vi "GetClassPath.vi"(8 "error in":errorcluster, 10 "class name":string, 11 "CEF_Repository in":refnum<class "CEF_Repository.lvclass">) -> (0 "error out":errorcluster, 2 "class path":path, 3 "CEF_Repository out":refnum<class "CEF_Repository.lvclass">)   [LabVIEW 2023, in "CEF.lvlib" / "CEF_Repository.lvclass"]
doc: "Gets the path to the Class based on the Class Name. \nThe default behavior is build the path of the class on top of the class folder path. The name of the class and the folder it contains needs to be the same. A simple lookup from index and name would be the other option.\nCopyright 2017 National Instruments Corporation\n\nLicensed under the Apache License, Version 2.0 (the \"License\"); you may not use this file except in compliance with the License. You may obtain a copy of the License at http://www.apache.org/licenses/LICENSE-2.0\nUnless required by applicable law or agreed to in writing, software distributed under the License is distributed on an \"AS IS\" BASIS, WITHOUT WARRANTIES OR CONDITIONS OF ANY KIND, either express or implied. See the License for the specific language governing permissions and limitations under the License."
uses:
  CEF_Repository.lvclass
  class discovery singleton/class discovery singleton methods.ctl
  CEF.lvlib
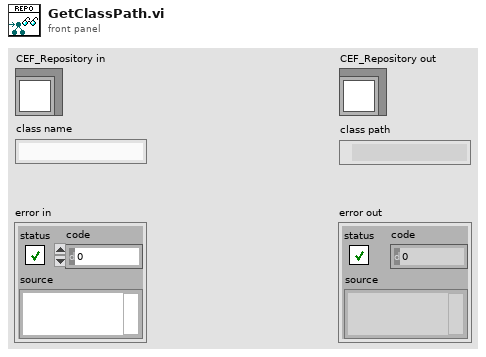
[diagram p1: front panel]
types:
  T1 = typedef "CEF.lvlib/class discovery singleton methods.ctl" = enum16{"add search paths", "load class by name", "list available classes", "get class path", "delete cache"}
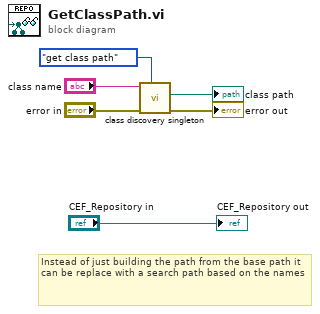
[diagram p0: block diagram]
diagram:
  # "Instead of just building the path from the base path it can be replace with a search path based on the names"
  n1 = call "class discovery singleton.vi"("method"=class_discovery_singleton_methods."get class path", "error in"="error in", "Class Name"="class name") -> ("error out"=→"error out":errorcluster, "class path"=→"class path":path)  [unwired: 5 in, 2 out]
  "CEF_Repository out" <- "CEF_Repository in"
